vi "test Script CD with Configuration.vi"(8 "error in":errorcluster, 11 "TestCase in":refnum<class "Scripting.lvclass">) -> (0 "error out":errorcluster, 3 "TestCase out":refnum<class "Scripting.lvclass">)   [LabVIEW 2020, in "Scripting.lvclass"]
uses:
  Scripting.lvclass
  <vilib>/addons/_JKI Toolkits/VI Tester/TestCase.llb/TestCase.lvclass
  Scripting/AIM MIL-STD-1553 Scripting.lvlib
  Shared/Address.ctl
  Shared/Message Type.ctl
  Shared/Terminal Endpoint.ctl
  Shared/Parameter Definition.ctl
  Shared/Message Definition.ctl
  Shared/1553 Channel.ctl
  Shared/Minor Frame Definition.ctl
  Shared/Major Frame Definition.ctl
  C:/dev/git/niveristand-custom-device-testing-tools/VeriStandScriptingTestCase/VeriStandScriptingTestCase.lvclass
  C:/Program Files (x86)/National Instruments/LabVIEW 2020/vi.lib/addons/_JKI Toolkits/VI Tester/TestCase.llb/TestCase.lvclass
  C:/dev/git/niveristand-aim-milStd1553-custom-device/Source/Custom Device Support/Tests/Unit/Scripting/Scripting.lvclass
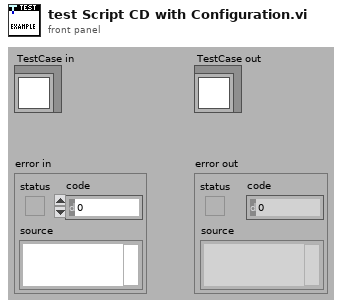
[diagram p1: front panel]
types:
  T1 = typedef "1553 Channel.ctl" = cluster{"HW channel":u16, "terminal addresses":T2[], "terminal names":string[], "acyclic frame names":string[], "major frames":T3[], "minor frames":T4[], "messages":T5[]}
  T2 = typedef "Address.ctl" = u16
  T3 = typedef "Major Frame Definition.ctl" = cluster{"name":string, "minor frames":string[]}
  T4 = typedef "Minor Frame Definition.ctl" = cluster{"name":string, "messages":string[]}
  T5 = typedef "Message Definition.ctl" = cluster{"name":string, "message type":T6, "endpoint Tx":T7, "endpoint Rx":T7, "create timestamp channel":bool, "mode code":u16, "number of words":u16, "parameters":cluster{"name":string, "default value":dbl, "unit":string, "parameter definition":T8}[]}
  T6 = typedef "Message Type.ctl" = string
  T7 = typedef "Terminal Endpoint.ctl" = cluster{"terminal address":T2, "subaddress":T2}
  T8 = typedef "Parameter Definition.ctl" = cluster{"start index":i32, "size (bits)":i32, "encoding":enum16{"BNR", "BCD", "Discrete"}, "signed":bool, "multiplier":dbl, "offset":dbl}
  T9 = typedef "Custom Device API.lvlib/Custom Device Item Ref.ctl" = u64
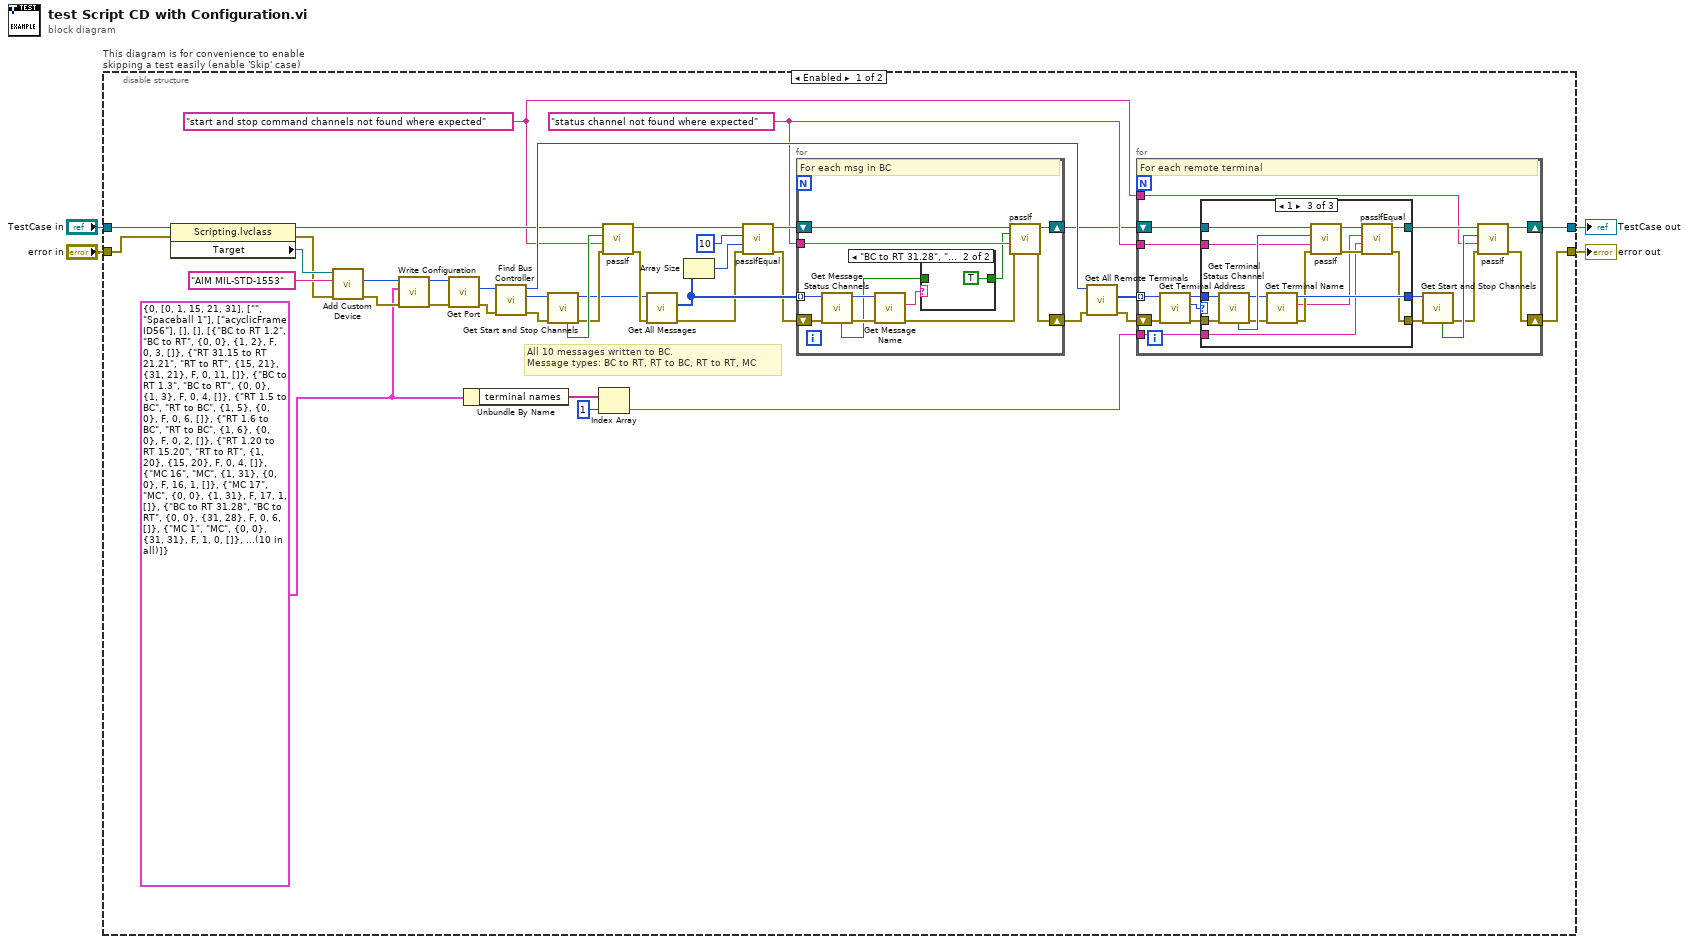
[diagram p0: block diagram]
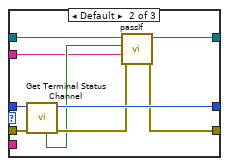
[diagram p4: hidden frame]
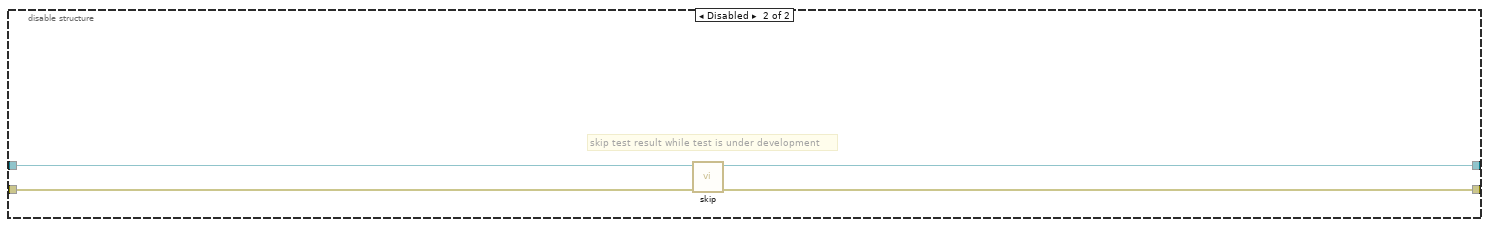
[diagram p5: hidden frame]
diagram:
  n1 = disable-structure "This diagram is for convenience to enable skipping a test easily (enable 'Skip' case)" shown="Enabled" {
    disable-tunnel: "TestCase in" -> [w41 w103]
    disable-tunnel: [w30 w101] -> w1
    disable-tunnel: [w29 w102] -> w3
    disable-tunnel: "error in" -> [w37 w100]
    frame Enabled {
      w9 = T1 {"HW channel"=0, "terminal addresses"=[0, 1, 15, 21, 31], "terminal names"=["", "Spaceball 1"], "acyclic frame names"=["acyclicFrame ID56"], "major frames"=[], "minor frames"=[], "messages"=[{"name"="BC to RT 1.2", "message type"="BC to RT", "endpoint Tx"={"terminal address"=0, "subaddress"=0}, "endpoint Rx"={"terminal address"=1, "subaddress"=2}, "create timestamp channel"=FALSE, "mode code"=0, "number of words"=3, "parameters"=[]}, {"name"="RT 31.15 to RT 21.21", "message type"="RT to RT", "endpoint Tx"={"terminal address"=15, "subaddress"=21}, "endpoint Rx"={"terminal address"=31, "subaddress"=21}, "create timestamp channel"=FALSE, "mode code"=0, "number of words"=11, "parameters"=[]}, {"name"="BC to RT 1.3", "message type"="BC to RT", "endpoint Tx"={"terminal address"=0, "subaddress"=0}, "endpoint Rx"={"terminal address"=1, "subaddress"=3}, "create timestamp channel"=FALSE, "mode code"=0, "number of words"=4, "parameters"=[]}, {"name"="RT 1.5 to BC", "message type"="RT to BC", "endpoint Tx"={"terminal address"=1, "subaddress"=5}, "endpoint Rx"={"terminal address"=0, "subaddress"=0}, "create timestamp channel"=FALSE, "mode code"=0, "number of words"=6, "parameters"=[]}, {"name"="RT 1.6 to BC", "message type"="RT to BC", "endpoint Tx"={"terminal address"=1, "subaddress"=6}, "endpoint Rx"={"terminal address"=0, "subaddress"=0}, "create timestamp channel"=FALSE, "mode code"=0, "number of words"=2, "parameters"=[]}, {"name"="RT 1.20 to RT 15.20", "message type"="RT to RT", "endpoint Tx"={"terminal address"=1, "subaddress"=20}, "endpoint Rx"={"terminal address"=15, "subaddress"=20}, "create timestamp channel"=FALSE, "mode code"=0, "number of words"=4, "parameters"=[]}, {"name"="MC 16", "message type"="MC", "endpoint Tx"={"terminal address"=1, "subaddress"=31}, "endpoint Rx"={"terminal address"=0, "subaddress"=0}, "create timestamp channel"=FALSE, "mode code"=16, "number of words"=1, "parameters"=[]}, {"name"="MC 17", "message type"="MC", "endpoint Tx"={"terminal address"=0, "subaddress"=0}, "endpoint Rx"={"terminal address"=1, "subaddress"=31}, "create timestamp channel"=FALSE, "mode code"=17, "number of words"=1, "parameters"=[]}, {"name"="BC to RT 31.28", "message type"="BC to RT", "endpoint Tx"={"terminal address"=0, "subaddress"=0}, "endpoint Rx"={"terminal address"=31, "subaddress"=28}, "create timestamp channel"=FALSE, "mode code"=0, "number of words"=6, "parameters"=[]}, {"name"="MC 1", "message type"="MC", "endpoint Tx"={"terminal address"=0, "subaddress"=0}, "endpoint Rx"={"terminal address"=31, "subaddress"=31}, "create timestamp channel"=FALSE, "mode code"=1, "number of words"=0, "parameters"=[]}]} ("1553 channel")
      w15 = "start and stop command channels not found where expected" ("name")
      w23 = "status channel not found where expected" ("name")
      # "All 10 messages written to BC.\nMessage types: BC to RT, RT to BC, RT to RT, MC"
      n2 = property class="Scripting.lvclass"(reference=w41, error in=w37) -> (reference out=w19:refnum<class "Scripting.lvclass">, error out=w36:errorcluster, "Target"=w40:refnum<k24>)
      n3 = call "Add Custom Device.vi"("error in"=w36, "name"="AIM MIL-STD-1553", "target in"=w40) -> ("error out"=w38:errorcluster, "Ballard MIL-STD 1553 custom device"=w39:T9)  [unwired: 6 in, 1 out]
      n4 = call "Write Configuration.vi"("error in"=w38, "1553 configuration"=w9, "custom device ref"=w39) -> ("error out"=w7:errorcluster, "custom device ref out"=w8:T9)  [unwired: 7 in]
      n5 = call "Get Port.vi"("error in"=w7, "custom device ref"=w8) -> ("error out"=w6:errorcluster, "port"=w5:T9)  [unwired: 7 in, 1 out]
      n6 = Unbundle By Name(w9) -> ("terminal names"=w12:string[])
      n7 = call "Find Bus Controller.vi"("error in"=w6, "port in"=w5) -> ("error out"=w17:errorcluster, "bus controller"=w14:T9, "port out"=w33:T9)  [unwired: 6 in, 1 out]
      n8 = call "Get Start and Stop Channels.vi"("error in"=w17, "terminal in"=w14) -> ("error out"=w20:errorcluster, "terminal out"=w13:T9, "found?"=w21:bool)  [unwired: 5 in, 2 out]
      n9 = Index Array(array=w12, index=1) -> (element=w10:string)
      n10 = call-dynamic "passIf.vi"("error in (no error)"=w20, "message (\"\")"=w15, "pass"=w21, "TestCase in"=w19) -> ("error out"=w16:errorcluster, "TestCase out"=w18:refnum<class "Scripting.lvclass">)  [unwired: 6 in]
      n11 = call "Get All Messages.vi"("error in"=w16, "port in"=w13) -> ("error out"=w27:errorcluster, "messages"=w28:T9[])  [unwired: 7 in, 1 out]
      n12 = Array Size(array=w28) -> (size(s)=w35:i32)
      n13 = call-dynamic "passIfEqual.vi"("error in (no error)"=w27, "y"=w35, "x"=10 ("size(s)"), "TestCase in"=w18) -> ("error out"=w26:errorcluster, "TestCase out"=w25:refnum<class "Scripting.lvclass">)  [unwired: 6 in]
      n14 = for {
        tunnel: w28 -> [w53] mode=indexing
        shift-right: [w50] -> w24
        shift-left: w26 -> [w54]
        shift-right: [w51] -> w22
        shift-left: w25 -> [w52]
        tunnel: w23 -> [w49]
        # "For each msg in BC"
        n15 = call "Get Message Status Channels.vi"("error in"=w54, "message in"=w53) -> ("error out"=w48:errorcluster, "message out"=w47:T9, "found?"=w43:bool)  [unwired: 6 in, 1 out]
        n16 = call "Get Message Name.vi"("error in"=w48, "message in"=w47) -> ("error out"=w46:errorcluster, "message name"=w45:string)  [unwired: 6 in, 2 out]
        n17 = case shown="\"BC to RT 31.28\", \"MC 1\"" w45 {
          tunnel: w43 -> [w55 _]
          tunnel: [w55 TRUE ("found?")] -> w44
          frame Default {
          }
          frame "BC to RT 31.28", "MC 1" {
          }
        }
        n18 = call-dynamic "passIf.vi"("error in (no error)"=w46, "message (\"\")"=w49, "pass"=w44, "TestCase in"=w52) -> ("error out"=w50:errorcluster, "TestCase out"=w51:refnum<class "Scripting.lvclass">)  [unwired: 6 in]
      }
      n19 = call "Get All Remote Terminals.vi"("error in"=w24, "port in"=w33) -> ("error out"=w31:errorcluster, "remote terminals"=w32:T9[])  [unwired: 7 in, 1 out]
      n20 = for {
        tunnel: w32 -> [w61] mode=indexing
        shift-right: [w69] -> w29
        shift-left: w31 -> [w63]
        shift-right: [w71] -> w30
        shift-left: w22 -> [w67]
        tunnel: w23 -> [w64]
        tunnel: w15 -> [w58]
        tunnel: w10 -> [w57]
        # "For each remote terminal"
        n21 = call "Get Terminal Address.vi"("error in"=w63, "remote terminal in"=w61) -> ("error out"=w60:errorcluster, "terminal address"=w59:T2, "remote terminal out"=w62:T9)  [unwired: 6 in, 1 out]
        n22 = case shown="1" w59 {
          tunnel: [w73 w84 w92] -> w68
          tunnel: w67 -> [w75 w83 w99]
          tunnel: [w75 w82 w89] -> w66
          tunnel: [w74 w80 w87] -> w65
          tunnel: w64 -> [_ w78 w97]
          tunnel: w62 -> [w73 w77 w96]
          tunnel: w60 -> [w74 w76 w95]
          tunnel: w57 -> [_ _ w85]
          frame 31 {
          }
          frame Default {
            n23 = call "Get Terminal Status Channel.vi"("error in"=w76, "terminal in"=w77) -> ("error out"=w81:errorcluster, "terminal out"=w84:T9, "found?"=w79:bool)  [unwired: 6 in, 1 out]
            n24 = call-dynamic "passIf.vi"("error in (no error)"=w81, "message (\"\")"=w78, "pass"=w79, "TestCase in"=w83) -> ("error out"=w80:errorcluster, "TestCase out"=w82:refnum<class "Scripting.lvclass">)  [unwired: 6 in]
          }
          frame 1 {
            n25 = call "Get Terminal Status Channel.vi"("error in"=w95, "terminal in"=w96) -> ("error out"=w94:errorcluster, "terminal out"=w93:T9, "found?"=w98:bool)  [unwired: 6 in, 1 out]
            n26 = call "Get Terminal Name.vi"("error in"=w94, "remote terminal in"=w93) -> ("error out"=w91:errorcluster, "terminal name"=w86:string, "remote terminal out"=w92:T9)  [unwired: 7 in]
            n27 = call-dynamic "passIf.vi"("error in (no error)"=w91, "message (\"\")"=w97, "pass"=w98, "TestCase in"=w99) -> ("error out"=w88:errorcluster, "TestCase out"=w90:refnum<class "Scripting.lvclass">)  [unwired: 6 in]
            n28 = call-dynamic "passIfEqual.vi"("error in (no error)"=w88, "y"=w85, "x"=w86, "TestCase in"=w90) -> ("error out"=w87:errorcluster, "TestCase out"=w89:refnum<class "Scripting.lvclass">)  [unwired: 6 in]
          }
        }
        n29 = call "Get Start and Stop Channels.vi"("error in"=w65, "terminal in"=w68) -> ("error out"=w70:errorcluster, "found?"=w72:bool)  [unwired: 5 in, 3 out]
        n30 = call-dynamic "passIf.vi"("error in (no error)"=w70, "message (\"\")"=w58, "pass"=w72, "TestCase in"=w66) -> ("error out"=w69:errorcluster, "TestCase out"=w71:refnum<class "Scripting.lvclass">)  [unwired: 6 in]
      }
    }
    frame Disabled {
      # "skip test result while test is under development"
      n31 = call <vilib>:"skip.vi"("error in (no error)"=w100, "TestCase in"=w103) -> ("error out"=w102:errorcluster, "TestCase out"=w101:refnum<class "Scripting.lvclass">)  [unwired: 8 in]
    }
  }
  "error out" <- w3
  "TestCase out" <- w1
